vi "Example Configuration.vi"() -> ()   [LabVIEW 2013]
uses:
  C:/tf/play/labview/Tinkerforge.dll
panel:
  in  "uid":string="63oL6P"
  in  "port":i32=4223
  in  "host":string="localhost"
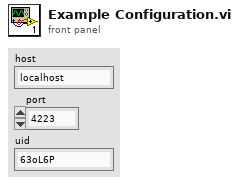
[diagram p1: front panel]
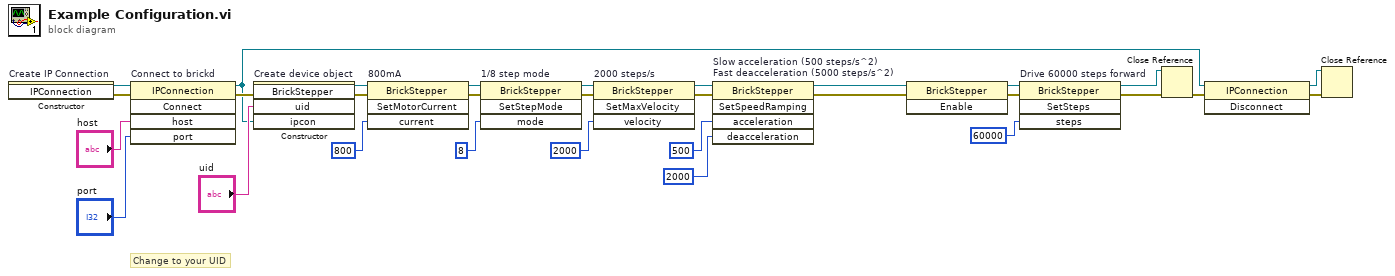
[diagram p0: block diagram]
diagram:
  # "Change to your UID"
  n1 = constructor on="Create IP Connection" class="IPConnection"() -> (reference out=w30:refnum<k24>, error out=w1:errorcluster)  [unwired: 3 in, 1 out]
  n2 = invoke on="Connect to brickd" class="IPConnection" method="Connect"(reference=w30, error in=w1, "host"="host", "port"="port") -> (reference out=w21:refnum<k24>, error out=w26:errorcluster)  [unwired: 1 in, 3 out]
  n3 = constructor on="Create device object" class="BrickStepper"(error in=w26, "uid"="uid", "ipcon"=w21) -> (reference out=w24:refnum<k24>, error out=w25:errorcluster)  [unwired: 2 in, 3 out]
  n4 = invoke on="800mA" class="BrickStepper" method="SetMotorCurrent"(reference=w24, error in=w25, "current"=800) -> (reference out=w16:refnum<k24>, error out=w18:errorcluster)  [unwired: 1 in, 2 out]
  n5 = invoke on="1/8 step mode" class="BrickStepper" method="SetStepMode"(reference=w16, error in=w18, "mode"=u8 8) -> (reference out=w15:refnum<k24>, error out=w17:errorcluster)  [unwired: 1 in, 2 out]
  n6 = invoke on="2000 steps/s" class="BrickStepper" method="SetMaxVelocity"(reference=w15, error in=w17, "velocity"=2000) -> (reference out=w11:refnum<k24>, error out=w12:errorcluster)  [unwired: 1 in, 2 out]
  n7 = invoke on="Slow acceleration (500 steps/s^2)\nFast deacceleration (5000 steps/s^2)" class="BrickStepper" method="SetSpeedRamping"(reference=w11, error in=w12, "acceleration"=500, "deacceleration"=2000) -> (reference out=w7:refnum<k24>, error out=w8:errorcluster)  [unwired: 1 in, 3 out]
  n8 = invoke class="BrickStepper" method="Enable"(reference=w7, error in=w8) -> (reference out=w5:refnum<k24>, error out=w6:errorcluster)  [unwired: 1 in, 1 out]
  n9 = invoke on="Drive 60000 steps forward" class="BrickStepper" method="SetSteps"(reference=w5, error in=w6, "steps"=60000) -> (reference out=w2:refnum<k24>, error out=w3:errorcluster)  [unwired: 1 in, 2 out]
  n10 = Close Reference(reference=w2, error in (no error)=w3) -> (error out=w23:errorcluster)
  n11 = invoke class="IPConnection" method="Disconnect"(reference=w21, error in=w23) -> (reference out=w20:refnum<k24>, error out=w22:errorcluster)  [unwired: 1 in, 1 out]
  n12 = Close Reference(reference=w20, error in (no error)=w22) -> ()  [unwired: 1 out]
